vi "poly_control_value_from_name_single.vi"(8 "error in (no error)":errorcluster, 10 "control name":string, 11 "vi ref":refnum<vi>) -> (0 "error out":errorcluster, 1 "Type":T1, 2 "Value":variant, 3 "vi ref dup":refnum<vi>, 4 "found?":bool, 5 "ctrl ref":refnum<vi>)   [LabVIEW 2015, in "_ref_tools_polys.lvlib"]
uses:
  _ref_tools_polys.lvlib
  <vilib>/Utility/Data Type/Type Definitions/Data Type.ctl
  <vilib>/Utility/Data Type/NI_Data Type.lvlib
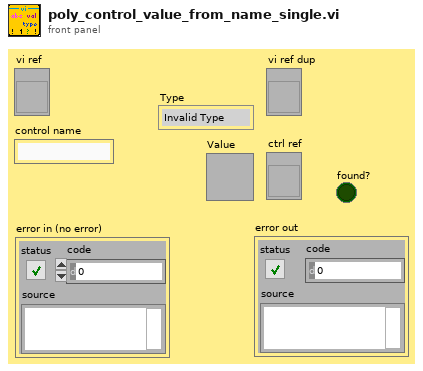
[diagram p1: front panel]
types:
  T1 = typedef "NI_Data Type.lvlib/Data Type.ctl" = enum8{"Invalid Type", "Void", "I8", "I16", "I32", "I64", "U8", "U16", "U32", "U64", "Single Float", "Double Float", "Extended Float", "Single Complex", "Double Complex", "Extended Complex", "Enum U8", "Enum U16", "Enum U32", "Enum U64", "Single Float With Unit", "Double Float With Unit", "Extended Float With Unit", "Single Complex with Unit", "Double Complex with Unit", "Extended Complex with Unit", "Boolean", "String", "Path", "Picture", "Tag", "Array", "Cluster", "Variant", "LV Variant", "Waveform", "Timestamp", "Digital Waveform", "Digital Data", "ExpressData", "Refnum", "External Data", "VI", "Poly VI", "LabVIEW Class Instance", "Fixed Point"}
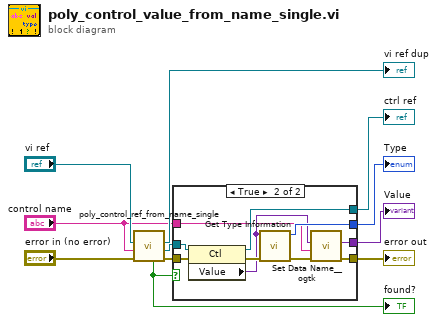
[diagram p0: block diagram]
diagram:
  n1 = call "poly_control_ref_from_name_single.vi"("error in (no error)"="error in (no error)", "control name"="control name", "vi ref"="vi ref") -> ("error out"=w4:errorcluster, "ctrl ref"=w8:refnum<vi>, "vi ref dup"=→"vi ref dup":refnum<vi>, "found?"=w2:bool)  [unwired: 5 in]
  "found?" <- w2
  n2 = case shown="True" w2 {
    tunnel: w8 -> [_ w22]
    tunnel: [_ w21] -> w7
    tunnel: [_ w14] -> w6
    tunnel: [_ w20] -> w5
    tunnel: w4 -> [w12 w19]
    tunnel: [w12 w16] -> w3
    tunnel: "control name" -> [_ w13]
    frame False {
    }
    frame True {
      n3 = property class="Ctl"(reference=w22, error in=w19) -> (reference out=w21:refnum<vi>, error out=w18:errorcluster, "Value"=w15:variant)
      n4 = call <vilib>:"Get Type Information.vi"("error in (no error)"=w18, "Variant"=w15) -> ("error out"=w17:errorcluster, "Type"=w20:T1)  [unwired: 5 in, 3 out]
      n5 = call <userlib>:"Set Data Name__ogtk.vi"("error in (no error)"=w17, "Data Name"=w13, "Data"=w15) -> ("error out"=w16:errorcluster, "Renamed Data"=w14:variant)  [unwired: 7 in]
    }
  }
  "ctrl ref" <- w7
  "error out" <- w3
  "Type" <- w5
  "Value" <- w6
